vi "thcd_get_chan.vi"(8 "err_in":errorcluster, 9 "thcd_ch":T1, 10 "thcd_delay":u32=500, 11 "thcd_visa":refnum<visa-resource-name>) -> (0 "res_4":T3 {"res_gid" items=["ERR", "1", "2", "C3H6O ", "C2H3N ", "C2H2 ", "Air ", "C3H4 ", "NH3 ", "Ar ", "AsH3 ", "C6H6 ", "BCl3 ", "BF3 ", "Br2 ", "15", "16", "CBrF3 ", "C4H10 ", "19", "C4H8 ", "CO2 ", "CS2 ", "CO ", "CCl4 ", "COS ", "Cl2 ", "ClF3 ", "28", "29", "CHCl3 ", "31", "32", "C4H8 ", "C2N2 ", "ClCN ", "C4H8 ", "C3H6 ", "H22 ", "B2H6 ", "40", "R21 ", "42", "43", "44", "45", "46", "47", "48", "C2H7N ", "C2H6O ", "C2H6S ", "C4H6 ", "C2H6 ", "54", "55", "C2H6O ", "C4H6 ", "C2H7N ", "C8H10 ", "60", "61", "C2H5F ", "C2H4 ", "64", "65", "C2H4O ", "C2H4N ", "68", "C2H6S ", "F2 ", "CH2O ", "CCl3F ", "73", "CClF3 ", "CF4 ", "76", "CHF3 ", "78", "C4H4O ", "He ", "C3HF7 ", "HMDS ", "83", "C6H14 ", "C6F6 ", "C6H12 ", "N2H4 ", "H2 ", "HBr ", "HCl ", "CHN ", "HF ", "HI ", "H2Se ", "H2S ", "C4H10 ", "97", "C4H8 ", "C5H12 ", "C 3H8O ", "101", "C 2H2O ", "Kr ", "CH4 ", "CH4O ", "106", "C3H4 ", "CH5N ", "CH3Br ", "CH3Cl ", "C7H14 ", "C3H9N ", "C 3H8O ", "C3H8S ", "CH3F ", "116", "CH3I ", "CH4S ", "C6H12 ", "C 3H6O ", "Ne ", "NO ", "N2 ", "NO2 ", "N2O4 ", "NF3 ", "127", "NOCl ", "N2O ", "C5H12 ", "C8H18 ", "O2 ", "F2O ", "O3 ", "B5H9 "]}, 1 "res_3":T3 {"res_gid" items=["ERR", "1", "2", "C3H6O ", "C2H3N ", "C2H2 ", "Air ", "C3H4 ", "NH3 ", "Ar ", "AsH3 ", "C6H6 ", "BCl3 ", "BF3 ", "Br2 ", "15", "16", "CBrF3 ", "C4H10 ", "19", "C4H8 ", "CO2 ", "CS2 ", "CO ", "CCl4 ", "COS ", "Cl2 ", "ClF3 ", "28", "29", "CHCl3 ", "31", "32", "C4H8 ", "C2N2 ", "ClCN ", "C4H8 ", "C3H6 ", "H22 ", "B2H6 ", "40", "R21 ", "42", "43", "44", "45", "46", "47", "48", "C2H7N ", "C2H6O ", "C2H6S ", "C4H6 ", "C2H6 ", "54", "55", "C2H6O ", "C4H6 ", "C2H7N ", "C8H10 ", "60", "61", "C2H5F ", "C2H4 ", "64", "65", "C2H4O ", "C2H4N ", "68", "C2H6S ", "F2 ", "CH2O ", "CCl3F ", "73", "CClF3 ", "CF4 ", "76", "CHF3 ", "78", "C4H4O ", "He ", "C3HF7 ", "HMDS ", "83", "C6H14 ", "C6F6 ", "C6H12 ", "N2H4 ", "H2 ", "HBr ", "HCl ", "CHN ", "HF ", "HI ", "H2Se ", "H2S ", "C4H10 ", "97", "C4H8 ", "C5H12 ", "C 3H8O ", "101", "C 2H2O ", "Kr ", "CH4 ", "CH4O ", "106", "C3H4 ", "CH5N ", "CH3Br ", "CH3Cl ", "C7H14 ", "C3H9N ", "C 3H8O ", "C3H8S ", "CH3F ", "116", "CH3I ", "CH4S ", "C6H12 ", "C 3H6O ", "Ne ", "NO ", "N2 ", "NO2 ", "N2O4 ", "NF3 ", "127", "NOCl ", "N2O ", "C5H12 ", "C8H18 ", "O2 ", "F2O ", "O3 ", "B5H9 "]}, 2 "res_2":T3 {"res_gid" items=["ERR", "1", "2", "C3H6O ", "C2H3N ", "C2H2 ", "Air ", "C3H4 ", "NH3 ", "Ar ", "AsH3 ", "C6H6 ", "BCl3 ", "BF3 ", "Br2 ", "15", "16", "CBrF3 ", "C4H10 ", "19", "C4H8 ", "CO2 ", "CS2 ", "CO ", "CCl4 ", "COS ", "Cl2 ", "ClF3 ", "28", "29", "CHCl3 ", "31", "32", "C4H8 ", "C2N2 ", "ClCN ", "C4H8 ", "C3H6 ", "H22 ", "B2H6 ", "40", "R21 ", "42", "43", "44", "45", "46", "47", "48", "C2H7N ", "C2H6O ", "C2H6S ", "C4H6 ", "C2H6 ", "54", "55", "C2H6O ", "C4H6 ", "C2H7N ", "C8H10 ", "60", "61", "C2H5F ", "C2H4 ", "64", "65", "C2H4O ", "C2H4N ", "68", "C2H6S ", "F2 ", "CH2O ", "CCl3F ", "73", "CClF3 ", "CF4 ", "76", "CHF3 ", "78", "C4H4O ", "He ", "C3HF7 ", "HMDS ", "83", "C6H14 ", "C6F6 ", "C6H12 ", "N2H4 ", "H2 ", "HBr ", "HCl ", "CHN ", "HF ", "HI ", "H2Se ", "H2S ", "C4H10 ", "97", "C4H8 ", "C5H12 ", "C 3H8O ", "101", "C 2H2O ", "Kr ", "CH4 ", "CH4O ", "106", "C3H4 ", "CH5N ", "CH3Br ", "CH3Cl ", "C7H14 ", "C3H9N ", "C 3H8O ", "C3H8S ", "CH3F ", "116", "CH3I ", "CH4S ", "C6H12 ", "C 3H6O ", "Ne ", "NO ", "N2 ", "NO2 ", "N2O4 ", "NF3 ", "127", "NOCl ", "N2O ", "C5H12 ", "C8H18 ", "O2 ", "F2O ", "O3 ", "B5H9 "]}, 3 "res":T3 {"res_gid" items=["ERR", "1", "2", "C3H6O ", "C2H3N ", "C2H2 ", "Air ", "C3H4 ", "NH3 ", "Ar ", "AsH3 ", "C6H6 ", "BCl3 ", "BF3 ", "Br2 ", "15", "16", "CBrF3 ", "C4H10 ", "19", "C4H8 ", "CO2 ", "CS2 ", "CO ", "CCl4 ", "COS ", "Cl2 ", "ClF3 ", "28", "29", "CHCl3 ", "31", "32", "C4H8 ", "C2N2 ", "ClCN ", "C4H8 ", "C3H6 ", "H22 ", "B2H6 ", "40", "R21 ", "42", "43", "44", "45", "46", "47", "48", "C2H7N ", "C2H6O ", "C2H6S ", "C4H6 ", "C2H6 ", "54", "55", "C2H6O ", "C4H6 ", "C2H7N ", "C8H10 ", "60", "61", "C2H5F ", "C2H4 ", "64", "65", "C2H4O ", "C2H4N ", "68", "C2H6S ", "F2 ", "CH2O ", "CCl3F ", "73", "CClF3 ", "CF4 ", "76", "CHF3 ", "78", "C4H4O ", "He ", "C3HF7 ", "HMDS ", "83", "C6H14 ", "C6F6 ", "C6H12 ", "N2H4 ", "H2 ", "HBr ", "HCl ", "CHN ", "HF ", "HI ", "H2Se ", "H2S ", "C4H10 ", "97", "C4H8 ", "C5H12 ", "C 3H8O ", "101", "C 2H2O ", "Kr ", "CH4 ", "CH4O ", "106", "C3H4 ", "CH5N ", "CH3Br ", "CH3Cl ", "C7H14 ", "C3H9N ", "C 3H8O ", "C3H8S ", "CH3F ", "116", "CH3I ", "CH4S ", "C6H12 ", "C 3H6O ", "Ne ", "NO ", "N2 ", "NO2 ", "N2O4 ", "NF3 ", "127", "NOCl ", "N2O ", "C5H12 ", "C8H18 ", "O2 ", "F2O ", "O3 ", "B5H9 "]}, 4 "thcd_res_str":string, 5 "thcd_st":bool, 6 "err_out":errorcluster, 7 "thcd_visa":refnum<visa-resource-name>)   [LabVIEW 2013]
uses:
  thcd_controls/ctrl_chn_thcd.ctl
  thcd_controls/ctrl_gid_thcd.ctl
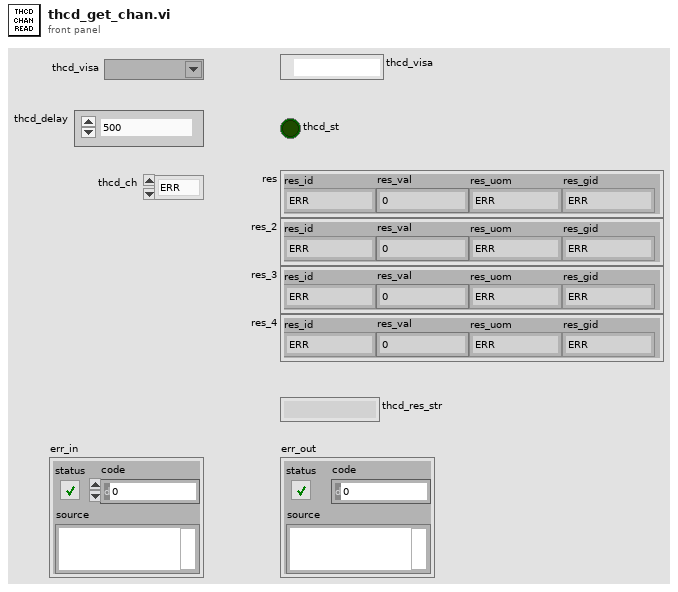
[diagram p1: front panel]
types:
  T1 = typedef "ctrl_chn_thcd.ctl" = enum8{"ERR", "1", "2", "3", "4", "ALL"}
  T2 = typedef "ctrl_gid_thcd.ctl" = u8
  T3 = cluster{"res_id":T1, "res_gid":T2, "res_uom":T1, "res_val":dbl}
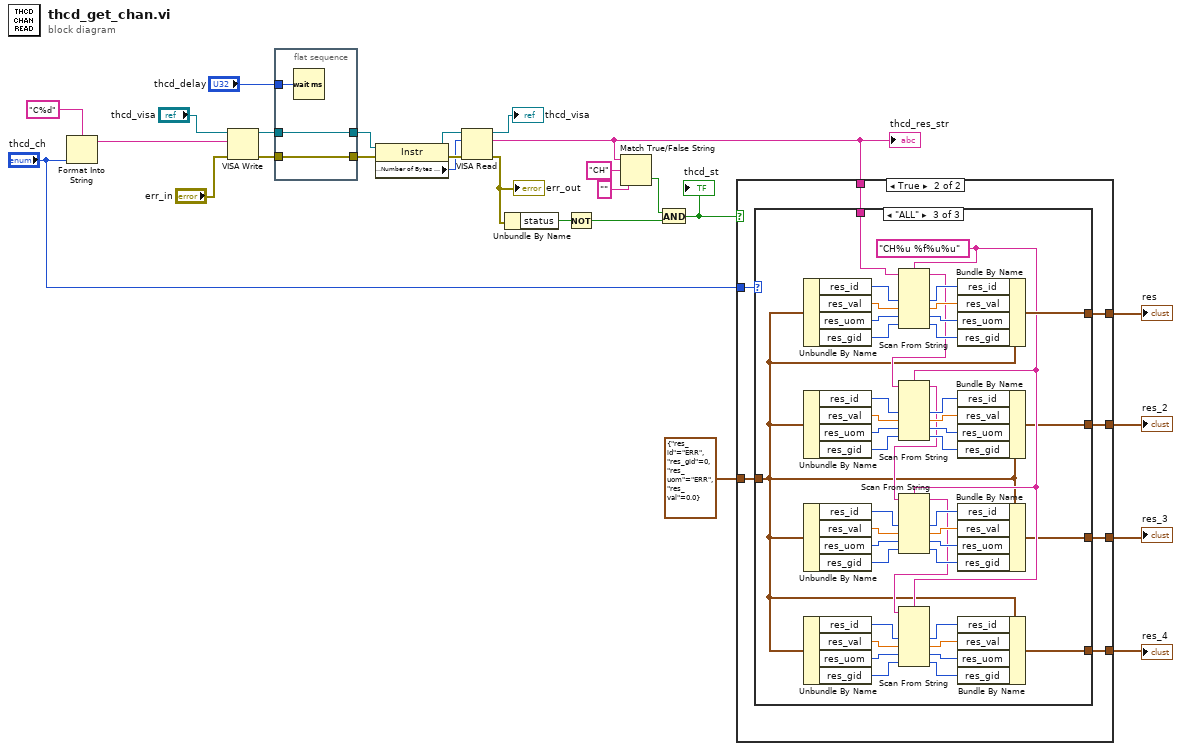
[diagram p0: block diagram]
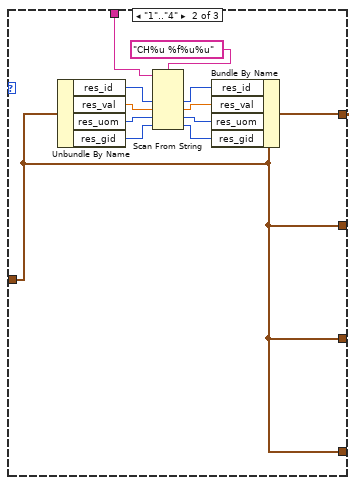
[diagram p4: hidden frame]
diagram:
  n1 = Format Into String(format string="C%d", "thcd_ch") -> (resulting string=w18:string)  [unwired: 2 in, 1 out]
  n2 = VISA Write(VISA resource name="thcd_visa", write buffer=w18, error in (no error)="err_in") -> (VISA resource name out=w25:refnum<visa-resource-name>, error out=w27:errorcluster)  [unwired: 1 out]
  n3 = flat-sequence {
    tunnel: w27 -> [w29]
    tunnel: [w29] -> w26
    tunnel: w25 -> [w28]
    tunnel: [w28] -> w24
    tunnel: "thcd_delay" -> [w30]
    frame #0 {
      n4 = Wait (ms)(milliseconds to wait=w30) -> ()  [unwired: 1 out]
    }
  }
  n5 = property class="Instr"(reference=w24, error in=w26) -> (reference out=w23:refnum<visa-resource-name>, error out=w22:errorcluster, "Serial Settings:Number of Bytes at Serial Port"=w10:u32)
  n6 = VISA Read(VISA resource name=w23, byte count=w10, error in (no error)=w22) -> (VISA resource name out=→"thcd_visa":refnum<visa-resource-name>, read buffer=w7:string, error out=w8:errorcluster)  [unwired: 1 out]
  "err_out" <- w8
  "thcd_res_str" <- w7
  n7 = Unbundle By Name(w8) -> ("status"=w4:bool)
  n8 = Not(x=w4) -> (.not. x?=w2:bool)
  n9 = Match True/False String(2:"" ("false string"), 3:"CH" ("true string"), 4:w7) -> (0:w3:bool)  [unwired: 1 out]
  n10 = And(x=w3, y=w2) -> (x .and. y?=w1:bool)
  "thcd_st" <- w1
  n11 = case shown="True" w1 {
    tunnel: "thcd_ch" -> [_ w38]
    tunnel: [w31 w37] -> w15
    tunnel: T3 {"res_id"=enum."ERR", "res_gid"=0, "res_uom"=enum."ERR", "res_val"=0.0} ("res 2") -> [w31 w36]
    tunnel: [w31 w35] -> w13
    tunnel: [w31 w34] -> w12
    tunnel: [w31 w33] -> w11
    tunnel: w7 -> [_ w32]
    frame False {
    }
    frame True {
      n12 = case shown="\"ALL\"" w38 {
        tunnel: w32 -> [_ w51 w93]
        tunnel: w36 -> [w39 w40 w55]
        tunnel: [w39 w46 w88] -> w37
        tunnel: [w39 w40 w54] -> w35
        tunnel: [w39 w40 w53] -> w34
        tunnel: [w39 w40 w52] -> w33
        frame Default {
        }
        frame "1".."4" {
          n13 = Unbundle By Name(w40) -> ("res_id"=w45:T1, "res_val"=w44:dbl, "res_uom"=w43:T1, "res_gid"=w42:T2)
          n14 = Scan From String(format string="CH%u %f%u%u" ("string"), input string=w51, default 1=w45, default 2=w44, default 3=w43, default 4=w42) -> (output 1=w50:T1, output 2=w49:dbl, output 3=w48:T1, output 4=w47:T2)  [unwired: 2 in, 3 out]
          n15 = Bundle By Name(cluster=w40, "res_id"=w50, "res_val"=w49, "res_uom"=w48, "res_gid"=w47) -> (w46:T3)
        }
        frame "ALL" {
          w56 = "CH%u %f%u%u" ("string")
          n16 = Unbundle By Name(w55) -> ("res_id"=w87:T1, "res_val"=w86:dbl, "res_uom"=w85:T1, "res_gid"=w84:T2)
          n17 = Unbundle By Name(w55) -> ("res_id"=w79:T1, "res_val"=w78:dbl, "res_uom"=w77:T1, "res_gid"=w76:T2)
          n18 = Unbundle By Name(w55) -> ("res_id"=w71:T1, "res_val"=w70:dbl, "res_uom"=w69:T1, "res_gid"=w68:T2)
          n19 = Unbundle By Name(w55) -> ("res_id"=w63:T1, "res_val"=w62:dbl, "res_uom"=w61:T1, "res_gid"=w60:T2)
          n20 = Scan From String(format string=w56, input string=w93, default 1=w87, default 2=w86, default 3=w85, default 4=w84) -> (remaining string=w59:string, output 1=w92:T1, output 2=w91:dbl, output 3=w90:T1, output 4=w89:T2)  [unwired: 2 in, 2 out]
          n21 = Scan From String(format string=w56, input string=w59, default 1=w79, default 2=w78, default 3=w77, default 4=w76) -> (remaining string=w58:string, output 1=w83:T1, output 2=w82:dbl, output 3=w81:T1, output 4=w80:T2)  [unwired: 2 in, 2 out]
          n22 = Scan From String(format string=w56, input string=w58, default 1=w71, default 2=w70, default 3=w69, default 4=w68) -> (remaining string=w57:string, output 1=w75:T1, output 2=w74:dbl, output 3=w73:T1, output 4=w72:T2)  [unwired: 2 in, 2 out]
          n23 = Scan From String(format string=w56, input string=w57, default 1=w63, default 2=w62, default 3=w61, default 4=w60) -> (output 1=w67:T1, output 2=w66:dbl, output 3=w65:T1, output 4=w64:T2)  [unwired: 2 in, 3 out]
          n24 = Bundle By Name(cluster=w55, "res_id"=w92, "res_val"=w91, "res_uom"=w90, "res_gid"=w89) -> (w88:T3)
          n25 = Bundle By Name(cluster=w55, "res_id"=w83, "res_val"=w82, "res_uom"=w81, "res_gid"=w80) -> (w54:T3)
          n26 = Bundle By Name(cluster=w55, "res_id"=w75, "res_val"=w74, "res_uom"=w73, "res_gid"=w72) -> (w53:T3)
          n27 = Bundle By Name(cluster=w55, "res_id"=w67, "res_val"=w66, "res_uom"=w65, "res_gid"=w64) -> (w52:T3)
        }
      }
    }
  }
  "res" <- w15
  "res_2" <- w13
  "res_3" <- w12
  "res_4" <- w11
